vi "Execute.Initialize.vi"(8 "error in (no error)":errorcluster, 11 "Cluster":T1={"NIVS.BaseLogPath"=path "", "NIVS.SystemDefinitionFile"=path "", "NIVS.Events"={"SequenceEvent"=refnum, "SystemChangeEvent"=refnum, "WorkspaceEvent"=refnum}, "NIVS.SequenceState"=enum."Idle", "NIVS.GatewayIPAddress"="", "NIVS.DataLogSpecRef"=refnum, "NIVS.DataLogManagerRef"=refnum, "NIVS.LogSessionGUID"="", "NIVS.WorkspaceManager"=refnum, "NIVS.Deployed"=FALSE, "NIVS.ProfileRef"=refnum, "NIVS.ProfileCallback"=refnum, "NIVS.SystemStateRefs"={"CustDatRef"=refnum, "EvtRef"=refnum}, "UI.Abort"=refnum, "UI.Pause"=refnum, "UI.EnableLogging"=refnum, "UI.Start"=refnum, "UI.LogChannels"=refnum, "UI.StartIteration"=refnum, "UI.StartStep"=refnum, "UI.Sequence"=refnum, "UI.PreviewMode"=refnum, "UI.Graph"=refnum, "UI.BaseFileName"=refnum, "UI.Profiles"=refnum, "UI.CurrentStep"=refnum, "UI.CurrentIteration"=refnum, "UI.TotalIterations"=refnum, "Sequence.AbortChannel"="", "Sequence.StepInfoChannel"="", "Sequence.Iterations"=0, "Sequence.IterationInfoChannel"="", "Sequence.#ofColumns"=0, "Events.State"=refnum, "Events.Test Result"=refnum, "Events.Progress"=refnum, "INI.Settings"={"Build Location"=path "C:/Simple Sequence Editor/SequenceRepo", "LoggingLocation"=path ""}}) -> (0 "error out":errorcluster)   [LabVIEW 2013, in "Simple Sequence Tools - Execution.lvlib"]
uses:
  Simple Sequence Tools - Execution.lvlib
  Types/Execuction.StateVariables.ctl
  Types/Execute.UserEventRefs.ctl
  <vilib>/NI Veristand/Execution/Workspace/SystemStateRegEventRef.ctl
  Types/Execution.SequenceState.ctl
  <vilib>/NI Veristand/Execution/DataLogging/DataLoggingSpecification Ref.ctl
  NationalInstruments.VeriStand.ClientAPI
  <vilib>/NI Veristand/Execution/DataLogging/IDataLogging Ref.ctl
  <vilib>/NI Veristand/Execution/Workspace/WorkspaceAPI.ctl
  NationalInstruments.VeriStand.RealTimeSequenceDefinitionApi
  <vilib>/NI Veristand/Execution/Workspace/SystemStateEventRef.ctl
  Shared/Types/INI.Settings
  Types/Execute.PreviewMode.ctl
  Shared/SubVIs/Constants.vi
  Shared/Simple Sequence Tools - Shared.lvlib
  <vilib>/NI Veristand/Execution/Workspace/NI_VS Workspace ExecutionAPI.lvlib
  <vilib>/NI Veristand/Execution/DataLogging/NI_VS Data Logging API.lvlib
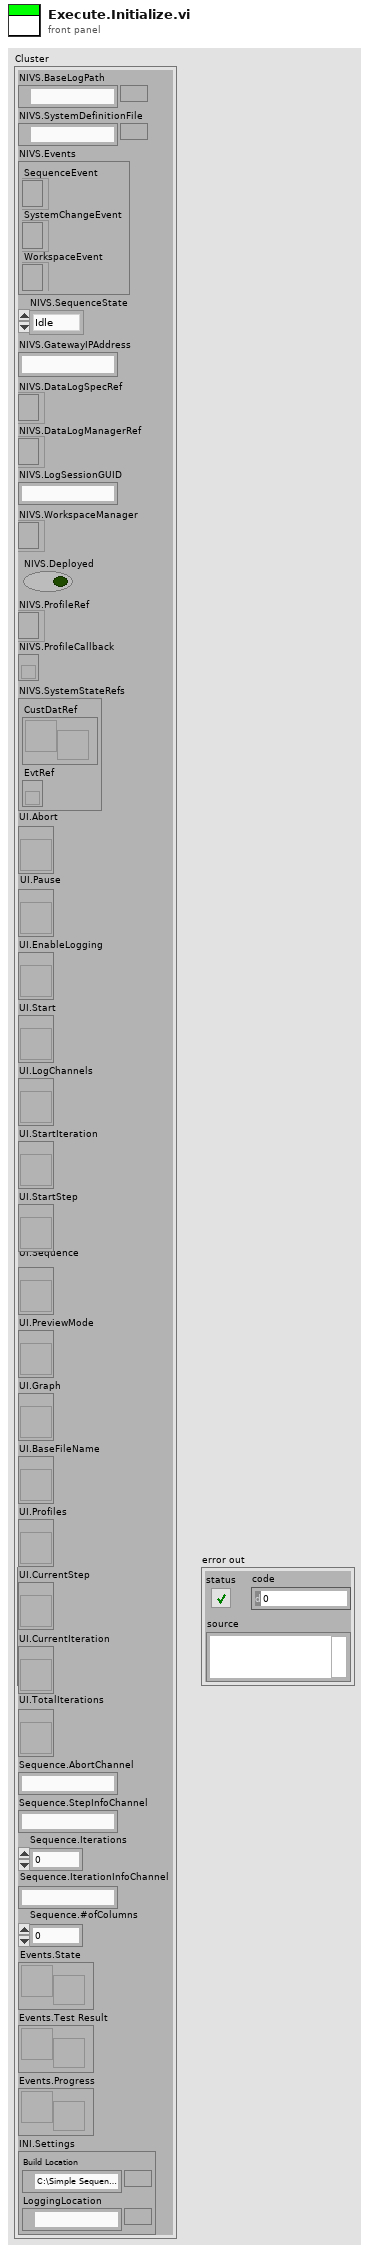
[diagram p1: front panel]
types:
  T1 = typedef "Simple Sequence Tools - Execution.lvlib/Execuction.StateVariables.ctl" = cluster{"NIVS.BaseLogPath":path, "NIVS.SystemDefinitionFile":path, "NIVS.Events":T2, "NIVS.SequenceState":T4, "NIVS.GatewayIPAddress":string, "NIVS.DataLogSpecRef":T5, "NIVS.DataLogManagerRef":T6, "NIVS.LogSessionGUID":string, "NIVS.WorkspaceManager":T7, "NIVS.Deployed":bool, "NIVS.ProfileRef":refnum<k24>, "NIVS.ProfileCallback":refnum<k27>, "NIVS.SystemStateRefs":T8, "UI.Abort":refnum<vi>, "UI.Pause":refnum<vi>, "UI.EnableLogging":refnum<vi>, "UI.Start":refnum<vi>, "UI.LogChannels":refnum<vi>, "UI.StartIteration":refnum<vi>, "UI.StartStep":refnum<vi>, "UI.Sequence":refnum<vi>, "UI.PreviewMode":refnum<vi>, "UI.Graph":refnum<vi>, "UI.BaseFileName":refnum<vi>, "UI.Profiles":refnum<vi>, "UI.CurrentStep":refnum<vi>, "UI.CurrentIteration":refnum<vi>, "UI.TotalIterations":refnum<vi>, "Sequence.AbortChannel":string, "Sequence.StepInfoChannel":string, "Sequence.Iterations":u32, "Sequence.IterationInfoChannel":string, "Sequence.#ofColumns":i32, "Events.State":refnum<user-event>, "Events.Test Result":refnum<user-event>, "Events.Progress":refnum<user-event>, "INI.Settings":T9}
  T2 = typedef "Simple Sequence Tools - Execution.lvlib/Execute.UserEventRefs.ctl" = cluster{"SequenceEvent":refnum<event-registration>, "SystemChangeEvent":T3, "WorkspaceEvent":refnum<event-registration>}
  T3 = typedef "NI_VS Workspace ExecutionAPI.lvlib/SystemStateRegEventRef.ctl" = refnum<event-registration>
  T4 = typedef "Simple Sequence Tools - Execution.lvlib/Execution.SequenceState.ctl" = enum16{"Idle", "Initializing", "Running", "Paused", "Finalizing", "Complete"}
  T5 = typedef "NI_VS Data Logging API.lvlib/DataLoggingSpecification Ref.ctl" = refnum<k24>
  T6 = typedef "NI_VS Data Logging API.lvlib/IDataLogging Ref.ctl" = refnum<k24>
  T7 = typedef "NI_VS Workspace ExecutionAPI.lvlib/WorkspaceAPI.ctl" = refnum<k24>
  T8 = typedef "NI_VS Workspace ExecutionAPI.lvlib/SystemStateEventRef.ctl" = cluster{"CustDatRef":refnum<user-event>, "EvtRef":refnum<k27>}
  T9 = typedef "Simple Sequence Tools - Shared.lvlib/INI.Settings" = cluster{"Build Location":path, "LoggingLocation":path}
  T10 = enum8{"Enabled", "Disabled", "Disabled and Grayed Out"}
  T11 = typedef "Simple Sequence Tools - Execution.lvlib/Execute.PreviewMode.ctl" = enum8{"Graph", "Table"}
  T12 = enum16{"Channels (No System Channel)", "Aliases", "All"}
  T13 = typedef "LVBoundsTypeDef.ctl" = cluster{"Width":u32, "Height":u32}
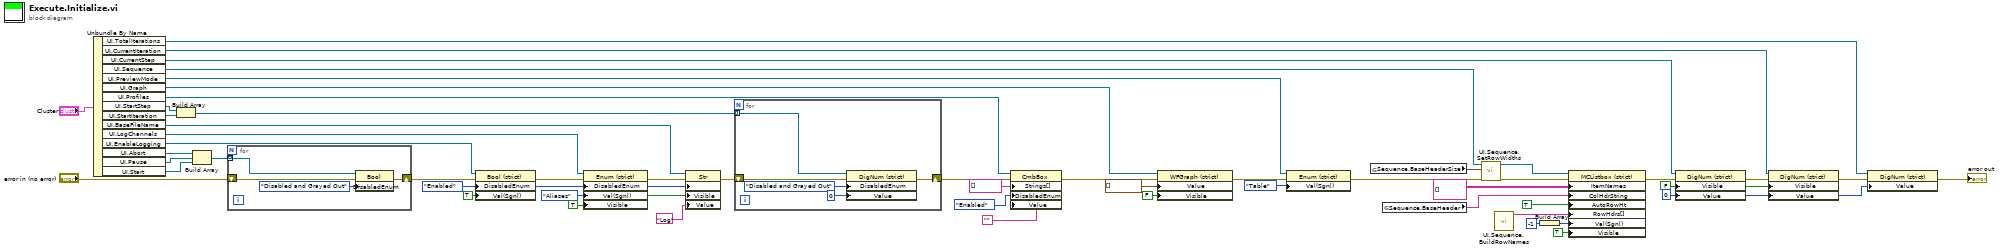
[diagram p0: block diagram]
diagram:
  w4 = u32 0 ("Value")
  w7 = FALSE ("Visible")
  w13 = TRUE ("Visible")
  w16 = T10."Enabled" ("Disabled")
  n1 = Unbundle By Name("Cluster") -> ("UI.TotalIterations"=w3:refnum<vi>, "UI.CurrentIteration"=w10:refnum<vi>, "UI.CurrentStep"=w11:refnum<vi>, "UI.Sequence"=w54:refnum<vi>, "UI.PreviewMode"=w41:refnum<vi>, "UI.Graph"=w38:refnum<vi>, "UI.Profiles"=w35:refnum<vi>, "UI.StartStep"=w32:refnum<vi>, "UI.StartIteration"=w31:refnum<vi>, "UI.BaseFileName"=w17:refnum<vi>, "UI.LogChannels"=w28:refnum<vi>, "UI.EnableLogging"=w27:refnum<vi>, "UI.Abort"=w22:refnum<vi>, "UI.Pause"=w23:refnum<vi>, "UI.Start"=w24:refnum<vi>)
  n2 = Build Array(w32, w31) -> (w33:refnum<vi>[])
  n3 = Build Array(w22, w23, w24) -> (w25:refnum<vi>[])
  n4 = for {
    tunnel: w25 -> [w58] mode=indexing
    shift-right: [w56] -> w26
    shift-left: "error in (no error)" -> [w55]
    n5 = property class="Bool"(reference=w58, error in=w55, "DisabledEnum"=T10."Disabled and Grayed Out" ("Disabled")) -> (error out=w56:errorcluster)  [unwired: 1 out]
  }
  n6 = property class="Bool (strict)"(reference=w27, error in=w26, "DisabledEnum"=w16, "Val(Sgnl)"=TRUE ("Value (Signaling)")) -> (error out=w29:errorcluster)  [unwired: 1 out]
  n7 = property class="Enum (strict)"(reference=w28, error in=w29, "DisabledEnum"=w16, "Val(Sgnl)"=T12."Aliases" ("Value (Signaling)"), "Visible"=w13) -> (error out=w15:errorcluster)  [unwired: 1 out]
  n8 = property class="Str"(reference=w17, error in=w15, "DisabledEnum"=w16, "Visible"=w13, "Value"="Log") -> (error out=w14:errorcluster)  [unwired: 1 out]
  n9 = for {
    tunnel: w33 -> [w63] mode=indexing
    shift-right: [w61] -> w34
    shift-left: w14 -> [w60]
    n10 = property class="DigNum (strict)"(reference=w63, error in=w60, "DisabledEnum"=T10."Disabled and Grayed Out" ("Disabled"), "Value"=u32 0) -> (error out=w61:errorcluster)  [unwired: 1 out]
  }
  n11 = property class="CmbBox"(reference=w35, error in=w34, "Strings[]"=string[] [] ("Strings []"), "DisabledEnum"=T10."Enabled" ("Disabled"), "Value"="") -> (error out=w37:errorcluster)  [unwired: 1 out]
  n12 = property class="WFGraph (strict)"(reference=w38, error in=w37, "Value"=waveform(dbl)[] [], "Visible"=FALSE) -> (error out=w42:errorcluster)  [unwired: 1 out]
  n13 = property class="Enum (strict)"(reference=w41, error in=w42, "Val(Sgnl)"=Execute.PreviewMode."Table" ("View")) -> (error out=w53:errorcluster)  [unwired: 1 out]
  n14 = global read "Constants.vi" "Sequence.BaseHeaderSize"() -> (w48:T13[])
  n15 = global read "Constants.vi" "Sequence.BaseHeader"() -> (w47:string[])
  n16 = call "UI.Sequence.SetRowWidths.vi"("error in (no error)"=w53, "CellSize"=w48, "UI.SequenceRef"=w54) -> ("error out"=w52:errorcluster, "UI.SequenceRef"=w45:refnum<vi>)  [unwired: 7 in]
  n17 = call "UI.Sequence.BuildRowNames.vi"() -> ("Row Headings"=w50:string[])  [unwired: 11 in]
  n18 = Build Array(-1 ("Value")) -> (w49:i32[])
  n19 = property class="MCListbox (strict)"(reference=w45, error in=w52, "ItemNames"=string[][] [] ("Item Names"), "ColHdrString"=w47, "AutoRowHt"=TRUE ("Autosizing Row Height"), "RowHdrs[]"=w50, "Val(Sgnl)"=w49, "Visible"=TRUE) -> (error out=w8:errorcluster)  [unwired: 1 out]
  n20 = property class="DigNum (strict)"(reference=w11, error in=w8, "Visible"=w7, "Value"=w4) -> (error out=w9:errorcluster)  [unwired: 1 out]
  n21 = property class="DigNum (strict)"(reference=w10, error in=w9, "Visible"=w7, "Value"=w4) -> (error out=w6:errorcluster)  [unwired: 1 out]
  n22 = property class="DigNum (strict)"(reference=w3, error in=w6, "Value"=w4) -> (error out=→"error out":errorcluster)  [unwired: 1 out]
